vi "Subtract float (single).vi"(8 "error in (no error)":errorcluster, 9 "y (0)":dbl, 10 "x (0)":dbl, 11 "XY-data in":cluster{"X-array":dbl[], "Y-array":dbl[]}) -> (0 "error out":errorcluster, 3 "XY-data out":cluster{"X-array":dbl[], "Y-array":dbl[]} {"Y-array" format="%.2p"; "X-array" format="%.2p"})   [LabVIEW 2016, in "xy_utilities.lvlib"]
uses:
  xy_utilities.lvlib
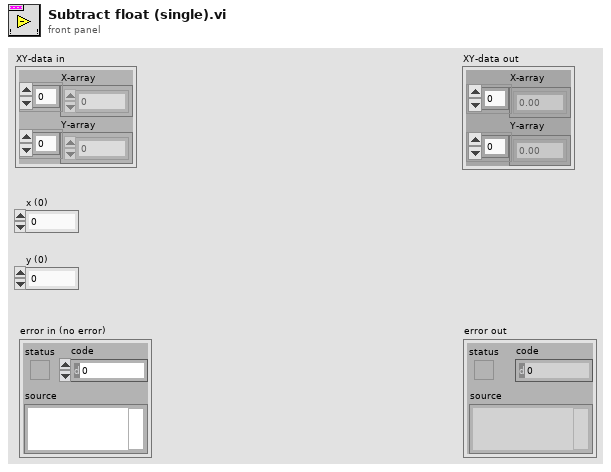
[diagram p1: front panel]
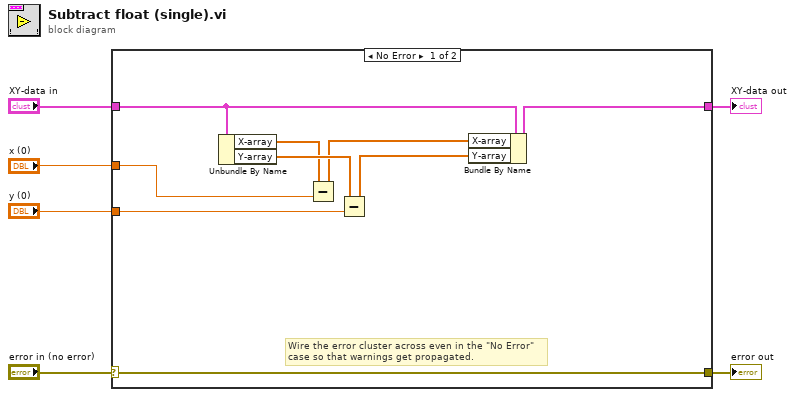
[diagram p0: block diagram]
diagram:
  n1 = case shown="No Error" "error in (no error)" {
    selector: "error in (no error)" -> [w15 w17]
    tunnel: [w15 w17] -> w5
    tunnel: "XY-data in" -> [w14 w16]
    tunnel: [w13 w16] -> w3
    tunnel: "y (0)" -> [w11 _]
    tunnel: "x (0)" -> [w7 _]
    frame No Error {
      # "Wire the error cluster across even in the \"No Error\"\ncase so that warnings get propagated."
      n2 = Unbundle By Name(w14) -> ("X-array"=w9:dbl[], "Y-array"=w12:dbl[])
      n3 = Subtract(x=w9, y=w7) -> (x-y=w8:dbl[])
      n4 = Subtract(x=w12, y=w11) -> (x-y=w10:dbl[])
      n5 = Bundle By Name(cluster=w14, "X-array"=w8, "Y-array"=w10) -> (w13:cluster{"X-array":dbl[], "Y-array":dbl[]})
    }
    frame Error {
    }
  }
  "error out" <- w5
  "XY-data out" <- w3
